vi "Get Water Level.vi"(8 "error in (no error)":errorcluster, 11 "Water Level in":refnum<class "Water Level.lvclass">) -> (0 "error out":errorcluster, 2 "Water Level":dbl)   [LabVIEW 2018, in "Water Level.lvlib" / "Water Level.lvclass"]
doc: "Child classes must override this method to return the depth of water in the water basin."
uses:
  Water Level.lvclass
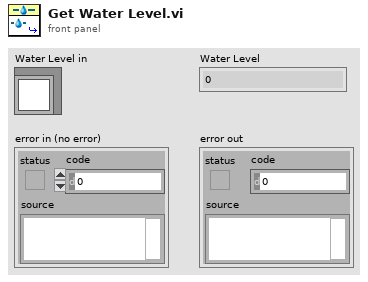
[diagram p1: front panel]
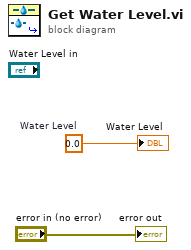
[diagram p0: block diagram]
diagram:
  w1 = 0.0  # Water Level
  "error out" <- "error in (no error)"
  "Water Level" <- w1
